vi "Read Data.vi"(4 "Length":u16, 5 "address":u32 format="%x", 6 "Time Out":u16=2000, 7 "bank":u8, 8 "error in (no error)":errorcluster, 10 "Baud Rate":u32=38400, 11 "COM Port":refnum<visa-resource-name>="COM4") -> (0 "error out":errorcluster, 1 "received str":string, 3 "Result":bool)   [LabVIEW 2018]
uses:
  RFID GlobalVariable.vi
panel:
  # "Data Read"
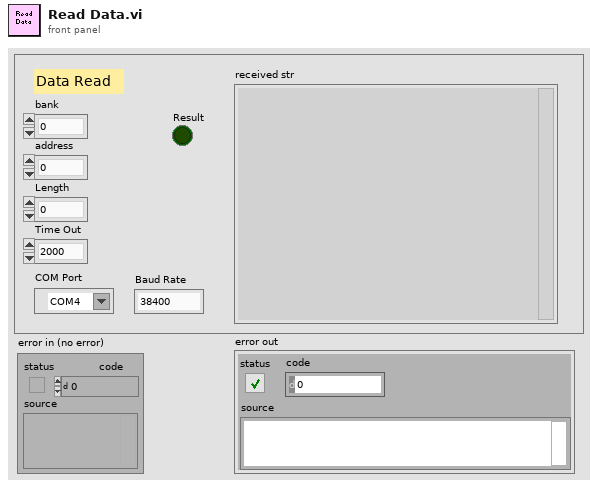
[diagram p1: front panel]
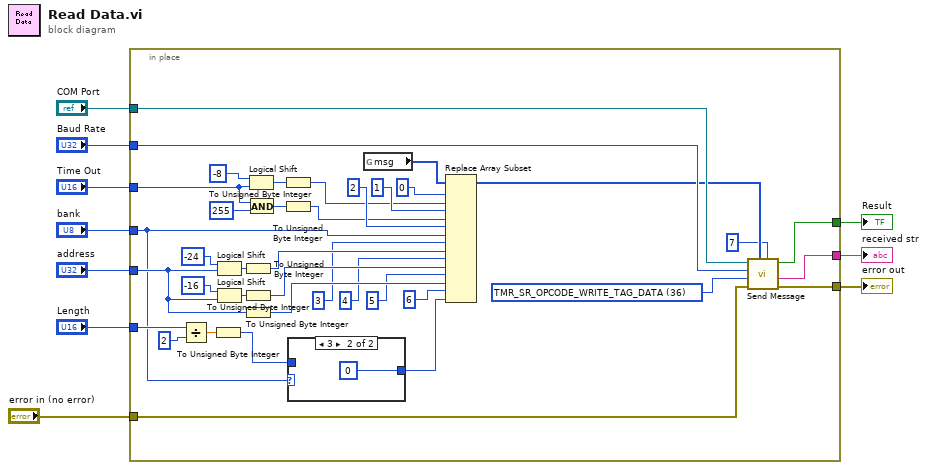
[diagram p0: block diagram]
diagram:
  n1 = in-place {
    in-place-border: "COM Port" -> [w48]
    in-place-border: "Baud Rate" -> [w47]
    in-place-border: "Time Out" -> [w46]
    in-place-border: "address" -> [w45]
    in-place-border: "Length" -> [w44]
    in-place-border: "bank" -> [w43]
    in-place-border: [w14] -> w4
    in-place-border: [w13] -> w3
    in-place-border: [w12] -> w2
    in-place-border: "error in (no error)" -> [w11]
    w42 = u16 36 items=["TMR_SR_OPCODE_VERSION"=3, "TMR_SR_OPCODE_SET_BAUD_RATE"=6, "TMR_SR_OPCODE_READ_TAG_ID_SINGLE"=33, "TMR_SR_OPCODE_READ_TAG_ID_MULTIPLE"=34, "TMR_SR_OPCODE_WRITE_TAG_ID"=35, "TMR_SR_OPCODE_WRITE_TAG_DATA"=36, "TMR_SR_OPCODE_KILL_TAG"=38, "TMR_SR_OPCODE_READ_TAG_DATA"=40, "TMR_SR_OPCODE_CLEAR_TAG_ID_BUFFER"=42, "TMR_SR_OPCODE_MULTI_PROTOCOL_TAG_OP"=47, "TMR_SR_OPCODE_GET_READ_TX_POWER"=98, "TMR_SR_OPCODE_GET_WRITE_TX_POWER"=100, "TMR_SR_OPCODE_GET_POWER_MODE"=104, "TMR_SR_OPCODE_GET_READER_OPTIONAL_PARAMS"=106, "TMR_SR_OPCODE_GET_PROTOCOL_PARAM"=107, "TMR_SR_OPCODE_SET_ANTENNA_PORT"=145, "TMR_SR_OPCODE_SET_TAG_PROTOCOL"=147, "TMR_SR_OPCODE_SET_READ_TX_POWER"=146, "TMR_SR_OPCODE_SET_WRITE_TX_POWER"=148, "TMR_SR_OPCODE_SET_REGION"=151, "TMR_SR_OPCODE_SET_READER_OPTIONAL_PARAMS"=154, "TMR_SR_OPCODE_SET_PROTOCOL_PARAM"=155] ("Opcode Constant")
    n2 = Divide(x=w44, y=u16 2) -> (x/y=w17:dbl)
    n3 = To Unsigned Byte Integer(number=w17) -> (unsigned 8bit integer=w16:u8)
    n4 = Logical Shift(y=i16 -24, x=w45) -> (x << y=w28:u32)
    n5 = Logical Shift(y=i16 -16, x=w45) -> (x << y=w27:u32)
    n6 = To Unsigned Byte Integer(number=w28) -> (unsigned 8bit integer=w25:u8)
    n7 = To Unsigned Byte Integer(number=w27) -> (unsigned 8bit integer=w24:u8)
    n8 = To Unsigned Byte Integer(number=w45) -> (unsigned 8bit integer=w23:u8)
    n9 = Logical Shift(y=i16 -8, x=w46) -> (x << y=w34:u16)
    n10 = And(x=w46, y=u16 255) -> (x .and. y?=w31:u16)
    n11 = To Unsigned Byte Integer(number=w34) -> (unsigned 8bit integer=w33:u8)
    n12 = To Unsigned Byte Integer(number=w31) -> (unsigned 8bit integer=w30:u8)
    n13 = case shown="3" w43 {
      tunnel: [w49 0] -> w15
      tunnel: w16 -> [w49 _]
      frame 0, Default {
      }
      frame 3 {
      }
    }
    n14 = global read "RFID GlobalVariable.vi" "msg"() -> (w41:u8[])
    n15 = Replace Array Subset(array=w41, new element #1=w33, index #1=0 ("index"), new element #2=w30, index #2=1 ("index"), new element #3=w43, index #3=2 ("index"), new element #4=w25, index #4=3 ("index"), new element #5=w24, index #5=4 ("index"), new element #6=w23, index #6=5 ("index"), new element #7=w15, index #7=6 ("index")) -> (w40:u8[])
    n16 = call "Send Message.vi"("Size"=u8 7, "Data"=w40, "error in (no error)"=w11, "Opcode"=w42, "Baud Rate"=w47, "COM Port"=w48) -> ("error out"=w12:errorcluster, "received str"=w14:string, "Result"=w13:bool)  [unwired: 2 in, 1 out]
  }
  "received str" <- w4
  "Result" <- w3
  "error out" <- w2
